vi "TDMS_Channel-Files_Config.vi"(8 "Error in":errorcluster caption="Fehler (Eingang, kein Fehler)", 9 "File operation (0:open)":T1(ring), 10 "File Names Array":string[](array[string]), 11 "stripped path":path) -> (0 "Error out":errorcluster caption="Fehler (Ausgang)", 2 "TDMS Write File Reference Array":refnum<k34>[](array[refnum]))   [LabVIEW 2016]
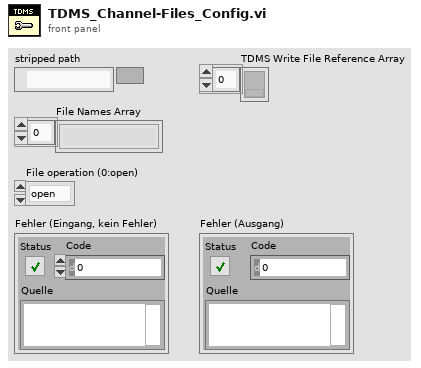
[diagram p1: front panel]
types:
  T1 = enum16{"open", "open or create", "create or replace", "create", "open (read-only)"}
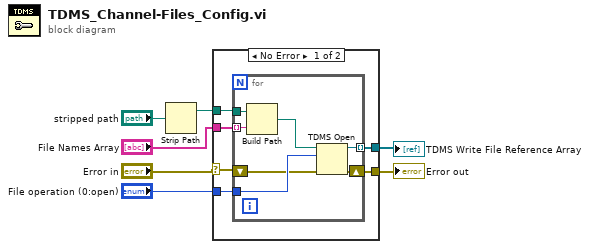
[diagram p0: block diagram]
diagram:
  n1 = Strip Path(path="stripped path") -> (stripped path=w2:path)  [unwired: 1 out]
  n2 = case shown="No Error" "Error in" {
    selector: "Error in" -> [w8 w21]
    tunnel: "File Names Array" -> [w13 _]
    tunnel: [w12 w21] -> w6
    tunnel: "File operation (0:open)" -> [w11 _]
    tunnel: [w10 _] -> w4
    tunnel: w2 -> [w9 _]
    frame No Error {
      n3 = for {
        tunnel: [w19] -> w10 mode=indexing
        tunnel: w13 -> [w18] mode=indexing
        tunnel: w11 -> [w17]
        tunnel: w9 -> [w16]
        shift-right: [w15] -> w12
        shift-left: w8 -> [w14]
        n4 = Build Path(base path=w16, name or relative path=w18) -> (appended path=w20:path)
        n5 = TDMS Open(8:w14, 10:w17, 11:w20) -> (0:w15:errorcluster, 3:w19:refnum<k34>)  [unwired: 4 in]
      }
    }
    frame Error {
    }
  }
  "Error out" <- w6
  "TDMS Write File Reference Array" <- w4
